vi "Target CSM.vi"(5 "Init State(\"Macro: Initialize\")":string="Macro: Initialize", 7 "Name (\"\" to Use UUID)":string="CSM Tiny") -> ()   [LabVIEW 2017]
doc: "Template for building CSM Module without User Interface.\n\n<b>Inputs:</b>\n- <b>Name (\"\" to Use UUID)</b>: Module Name\n - If Input is \"\", an uuid will be used for module name. The module is marked as stand-alone mode and will not be included in module list.\n - Fi Input end with '#', the module will worked in worker mode. Modules with the same name will shared the same message queue. Any external message will be processed by one of the modules, depends on who is free.\n - Otherwise, the input string will be used as module name, which should be unique in system. CSM will go to \"Critical Error\" state if duplicated module name is used in system.\n\n<b>Outputs:</b>\n - N/A"
uses:
  src/user.lib/_NEVSTOP/Communicable State Machine(CSM)/AdvanceAPI/CSM - Revert Arguments-Safe String.vi
  src/user.lib/_NEVSTOP/Communicable State Machine(CSM)/AdvanceAPI/CSM - Break Down Multiple States String.vi
  src/user.lib/_NEVSTOP/Communicable State Machine(CSM)/AdvanceAPI/CSM - Compact Multiple States.vi
  src/user.lib/_NEVSTOP/Communicable State Machine(CSM)/AdvanceAPI/CSM - Make String Arguments Safe.vi
  src/user.lib/_NEVSTOP/Communicable State Machine(CSM)/AdvanceAPI/CSM - Keywords.vi
  src/user.lib/_NEVSTOP/Communicable State Machine(CSM)/_Shared/Trim Single-line Text.vi
  src/user.lib/_NEVSTOP/Communicable State Machine(CSM)/Communicable State Machine.lvlib
panel:
  out "Error Occurred":errorcluster
  out "State History":string
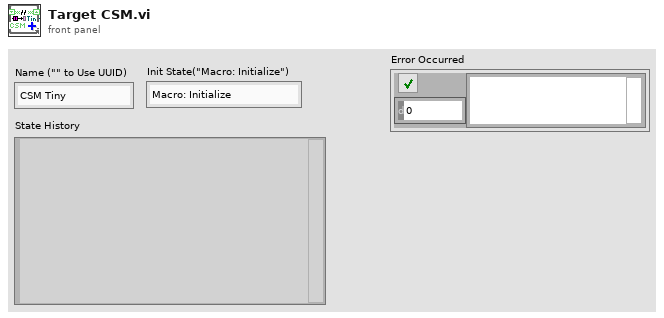
[diagram p1: front panel]
types:
  T1 = enum32{"Invalid", "Standard", "Closed", "Hidden", "Minimized", "Maximized"}
  T2 = enum32{"invalid app kind", "Development System", "Run Time System", "Student Edition", "Embedded LabVIEW", "Evaluation", "Custom"}
  T3 = typedef "Communicable State Machine.lvlib/_CSM_Response Source Message.ctl" = cluster{"‘State":string, "’Arguments":string, "’Error":errorcluster}
  T4 = cluster{"Current VI Reference":refnum<vi>, "Close Panel on Exit?":bool}
  T5 = cluster{"Core":cluster{"Current VI Reference":refnum<vi>, "Close Panel on Exit?":bool}, "Your Boolean data":bool, "Your string data":string}
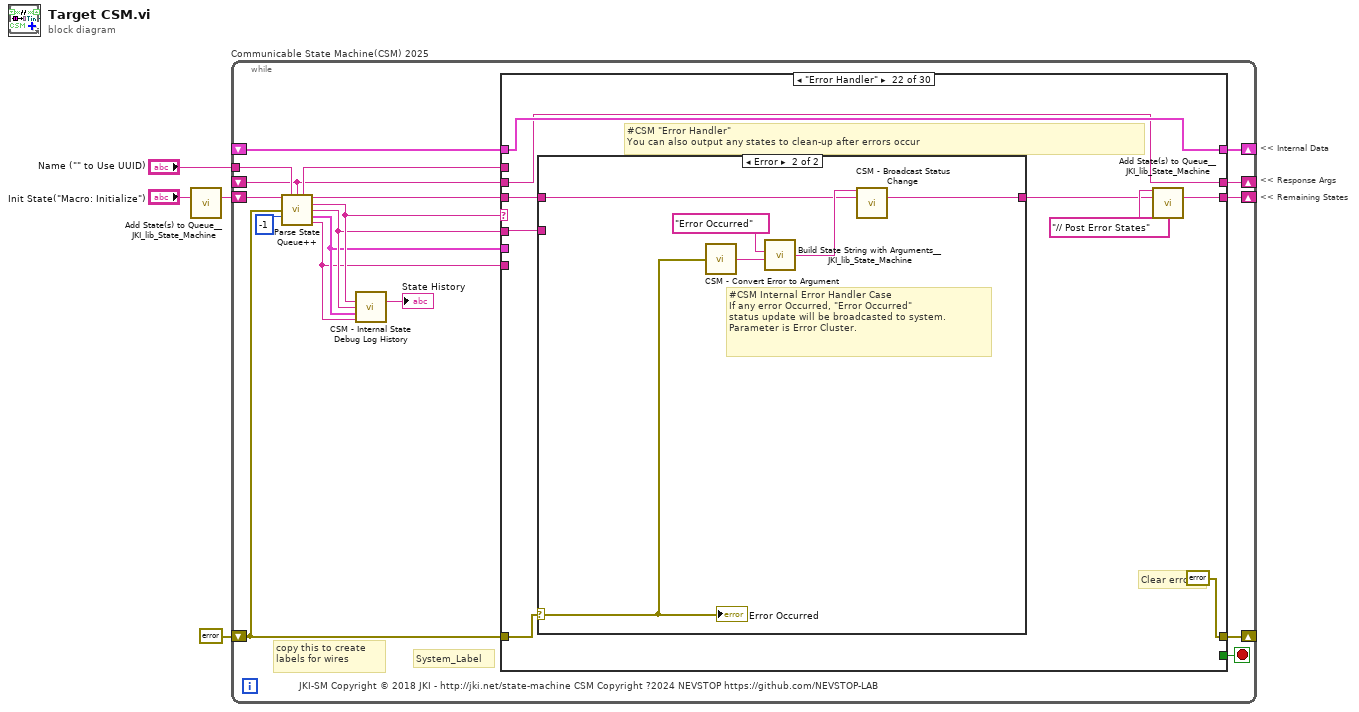
[diagram p0: block diagram]
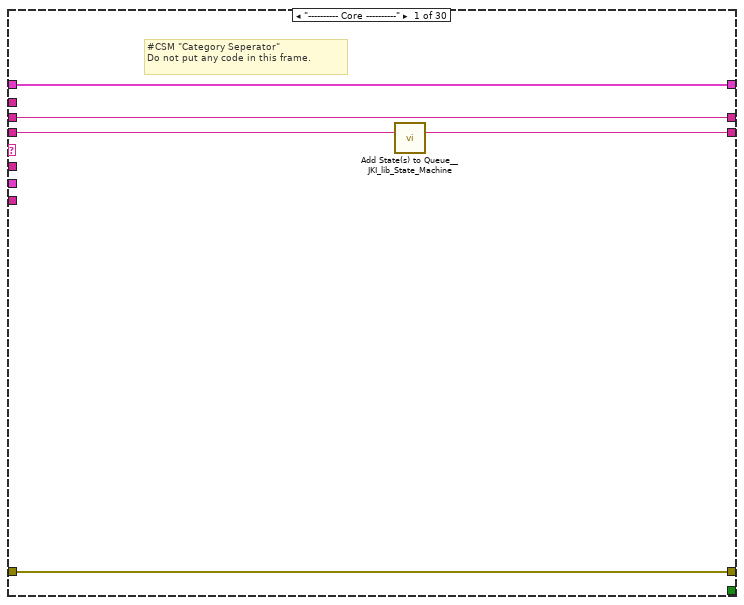
[diagram p2: hidden frame]
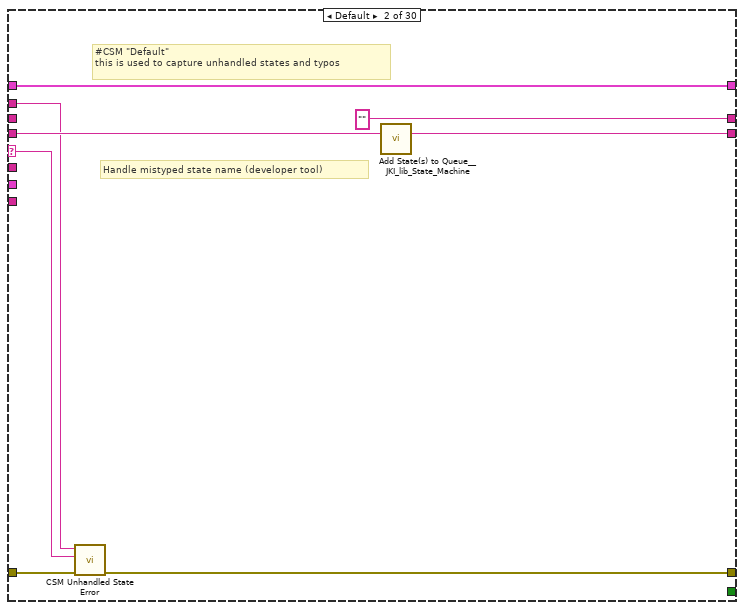
[diagram p3: hidden frame]
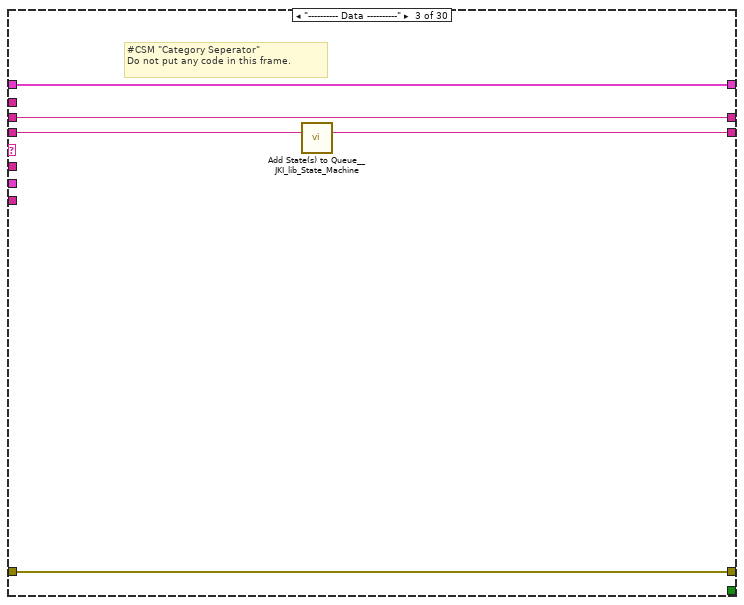
[diagram p4: hidden frame]
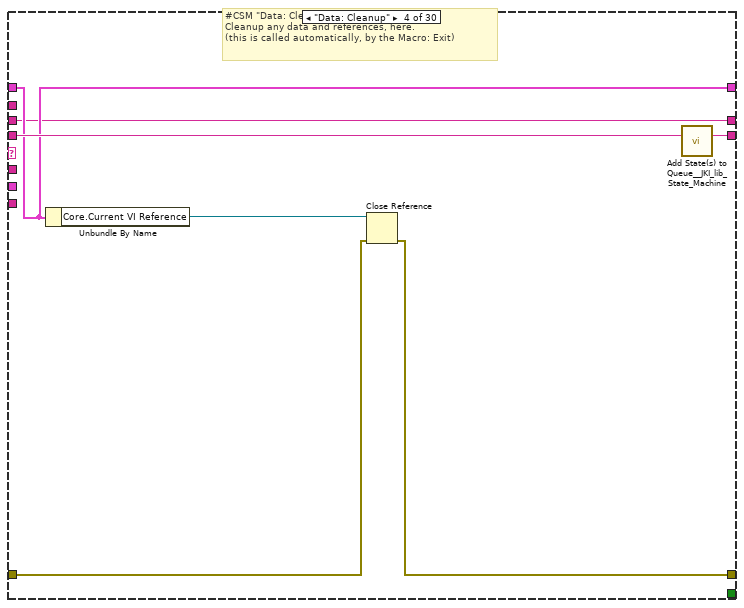
[diagram p5: hidden frame]
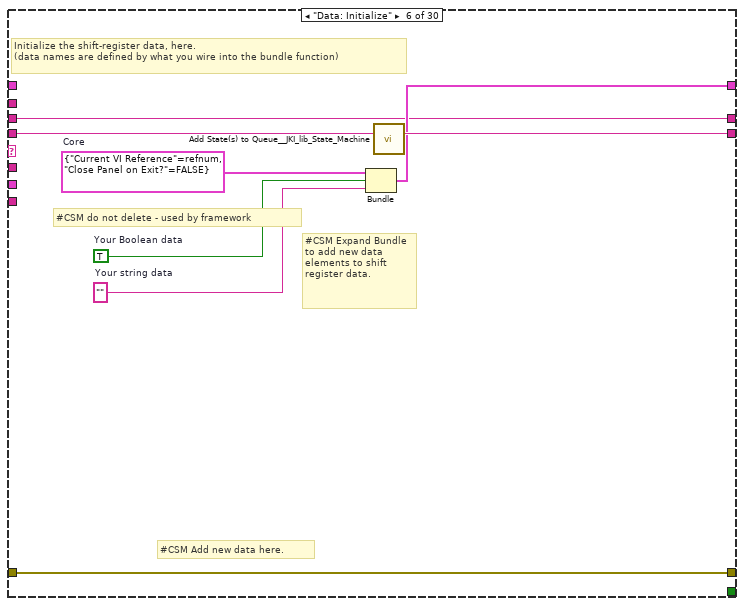
[diagram p7: hidden frame]
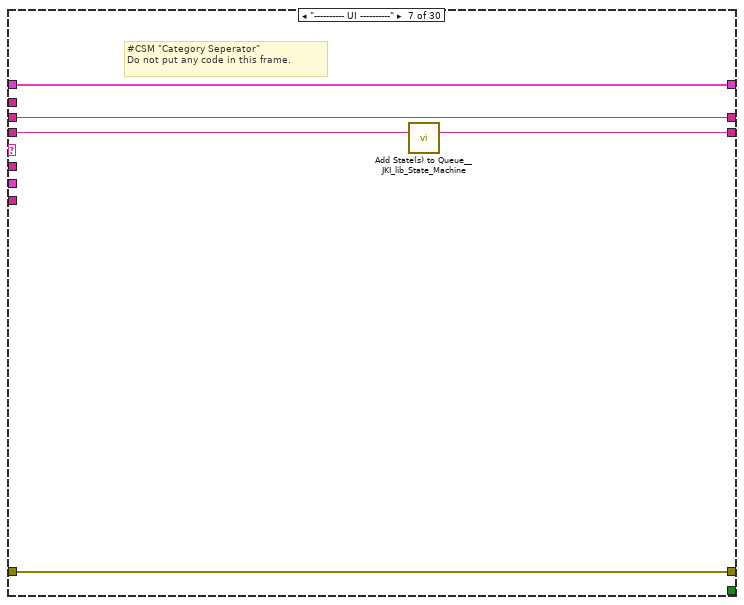
[diagram p8: hidden frame]
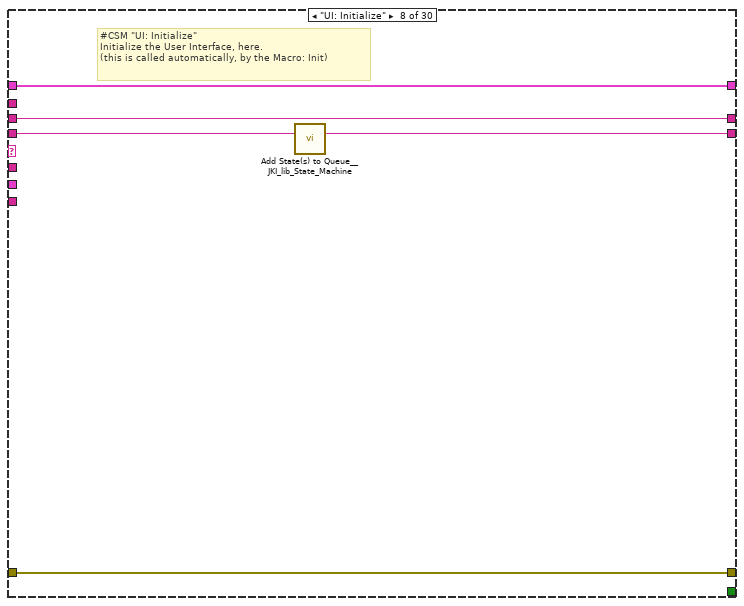
[diagram p9: hidden frame]
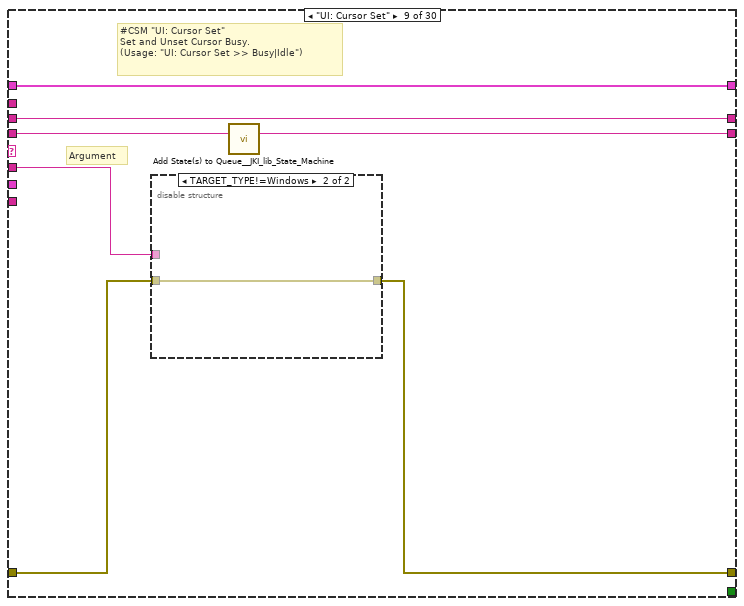
[diagram p10: hidden frame]
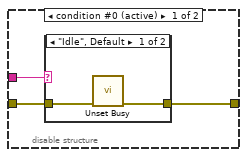
[diagram p11: hidden frame]
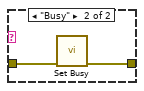
[diagram p12: hidden frame]
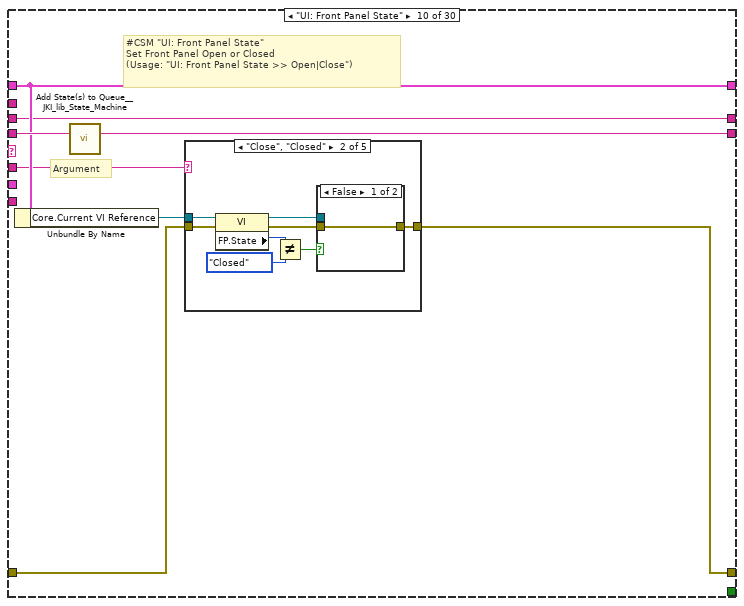
[diagram p13: hidden frame]
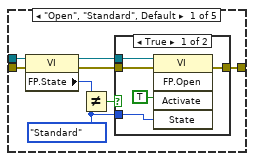
[diagram p14: hidden frame]
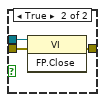
[diagram p16: hidden frame]
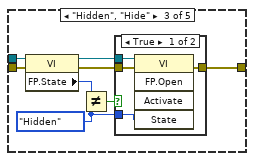
[diagram p17: hidden frame]
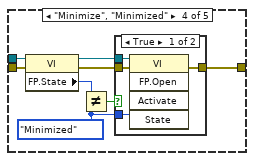
[diagram p19: hidden frame]
diagram:
  # "<< Internal Data"
  # "<< Response Args"
  # "<< Remaining States"
  n1 = call <vilib>:"Add State(s) to Queue__JKI_lib_State_Machine.vi"("State(s) in (\"\")"="Init State(\"Macro: Initialize\")") -> ("States Out"=w4:string)  [unwired: 14 in]
  n2 = while "Communicable State Machine(CSM) 2025" {
    shift-right: [w17] -> _
    shift-left: _ -> [w16]
    shift-right: [w20] -> _
    shift-left: errorcluster {"status"=FALSE, "code"=0, "source"=""} ("error out") -> [w15]
    shift-right: [w19] -> _
    shift-left: w4 -> [w21]
    tunnel: "Name (\"\" to Use UUID)" -> [w13]
    shift-right: [w14] -> _
    shift-left: _ -> [w7]
    stop <- w18 stop-if-true
    # "copy this to create labels for wires"
    # "System_Label"
    # "JKI-SM Copyright © 2018 JKI - http://jki.net/state-machine CSM Copyright ?2024 NEVSTOP https://github.com/NEVSTOP-LAB"
    n3 = call "Parse State Queue++.vi"("State Queue"=w21, "Name (\"\" to Use UUID)"=w13, "Response Arguments"=w7, "Previous Error"=w15, "Dequeue (1 ms)"=-1 ("Timeout")) -> ("Name Used"=w8:string, "Remaining States"=w22:string, "Current State"=w12:string, "Arguments"=w11:string, "Additional Information"=w10:T3, "Source CSM"=w9:string)  [unwired: 5 in]
    n4 = call "CSM - Internal State Debug Log History.vi"("State"=w12, "Arguments (\"\")"=w11, ">> Response Source Message >>"=w10, "Source (\"\")"=w9) -> ("Debug Log"=→"State History":string)  [unwired: 11 in]
    n5 = case shown="\"Error Handler\"" w12 {
      selector: w12 -> [_ w30 _ _ _ _ _ _ _ _ _ _ _ _ _ _ _ _ _ _ _ _ _ _ _ _ _ _ _ _]
      tunnel: w22 -> [w27 w34 w40 w47 w50 w59 w64 w69 w76 w92 w162 w170 w176 w179 w183 w189 w196 w201 w206 w209 w213 w219 w240 w247 w254 w265 w281 w289 w304 w310]
      tunnel: w11 -> [_ _ _ _ _ _ _ _ w71 w86 _ _ _ _ w185 _ _ _ _ _ _ w218 w239 w246 w253 w260 w276 _ _ _]
      tunnel: w16 -> [w24 w32 w37 w43 w51 _ w61 w67 w74 w88 w159 w165 w173 w178 w184 w190 w193 w199 w204 w210 w214 w216 w234 w242 w249 w263 w279 w290 w298 w308]
      tunnel: [w25 w28 w38 w44 w49 w56 w62 w66 w72 w89 w160 w164 w172 w180 w182 w188 w194 w198 w203 w208 w212 errorcluster {"status"=FALSE, "code"=0, "source"=""} ("error out") w236 w244 w251 w266 w282 w288 w292 w307] -> w20
      tunnel: w15 -> [w25 w35 w38 w45 w49 w56 w62 w66 w73 w90 w160 w164 w172 w180 w182 w188 w194 w198 w203 w208 w212 w217 w237 w245 w252 _ _ w288 w292 w307]
      tunnel: [w26 w33 w39 w42 w50 w58 w63 w68 w75 w91 w161 w169 w175 w179 w183 w189 w195 w200 w205 w209 w213 w220 w235 w243 w250 w264 w280 w289 w303 w309] -> w19
      tunnel: [_ _ _ _ _ _ _ _ _ _ _ _ _ _ _ _ _ _ _ _ _ _ _ _ _ _ _ _ _ TRUE] -> w18
      tunnel: [w24 w32 w37 w43 w51 w57 w61 w67 w74 w88 w159 w165 w173 w178 w184 w190 w193 w199 w204 w210 w214 w216 w234 w242 w249 w262 w278 w290 w302 w308] -> w17
      tunnel: w9 -> [_ _ _ _ _ _ _ _ _ _ _ _ _ _ _ _ _ _ _ _ _ _ _ _ _ w261 w277 _ _ _]
      tunnel: w10 -> [_ _ _ _ _ _ _ _ _ _ _ _ _ _ _ _ _ _ _ _ _ _ _ _ _ w256 w272 _ _ _]
      tunnel: [w23 "" w36 w41 w48 w52 w60 w65 w70 w85 w158 w163 w171 w177 w181 "API1 Response" w192 w197 w202 w207 w211 w215 w233 w241 w248 w255 w271 w287 w291 w306] -> w14
      tunnel: w8 -> [_ w29 _ _ _ _ _ _ _ _ _ _ _ _ _ _ _ _ _ _ _ _ w238 _ _ _ _ _ _ _]
      tunnel: w7 -> [w23 _ w36 w41 w48 w52 w60 w65 w70 w85 w158 w163 w171 w177 w181 _ w192 w197 w202 w207 w211 w215 w233 w241 w248 w255 w271 w287 w291 w306]
      frame "---------- Core ----------" {
        # "#CSM \"Category Seperator\"\nDo not put any code in this frame."
        n6 = call <vilib>:"Add State(s) to Queue__JKI_lib_State_Machine.vi"("State(s) in (\"\")"=w27) -> ("States Out"=w26:string)  [unwired: 14 in]
      }
      frame Default {
        # "#CSM \"Default\"\nthis is used to capture unhandled states and typos"
        # "Handle mistyped state name (developer tool)"
        n7 = call "CSM Unhandled State Error.vi"("error in (no error)"=w35, "Undefined State"=w30, "CSM Name"=w29) -> ("error out"=w28:errorcluster)  [unwired: 8 in]
        n8 = call <vilib>:"Add State(s) to Queue__JKI_lib_State_Machine.vi"("State(s) in (\"\")"=w34) -> ("States Out"=w33:string)  [unwired: 14 in]
      }
      frame "---------- Data ----------" {
        # "#CSM \"Category Seperator\"\nDo not put any code in this frame."
        n9 = call <vilib>:"Add State(s) to Queue__JKI_lib_State_Machine.vi"("State(s) in (\"\")"=w40) -> ("States Out"=w39:string)  [unwired: 14 in]
      }
      frame "Data: Cleanup" {
        # "#CSM \"Data: Cleanup\"\nCleanup any data and references, here.\n(this is called automatically, by the Macro: Exit)"
        n10 = Unbundle By Name(w43) -> ("Core.Current VI Reference"=w46:refnum<vi>)
        n11 = Close Reference(reference=w46, error in (no error)=w45) -> (error out=w44:errorcluster)
        n12 = call <vilib>:"Add State(s) to Queue__JKI_lib_State_Machine.vi"("State(s) in (\"\")"=w47) -> ("States Out"=w42:string)  [unwired: 14 in]
      }
      frame "Data: Update Indicators" {
      }
      frame "Data: Initialize" {
        w53 = T4 {"Current VI Reference"=refnum, "Close Panel on Exit?"=FALSE}  # Core
        w55 = TRUE  # Your Boolean data
        w54 = ""  # Your string data
        # "#CSM do not delete - used by framework"
        # "#CSM Expand Bundle to add new data elements to shift register data."
        # "#CSM Add new data here."
        # "Initialize the shift-register data, here.\n(data names are defined by what you wire into the bundle function)"
        n13 = Bundle("Core"=w53, "Your Boolean data"=w55, "Your string data"=w54) -> (w57:T5)  [unwired: 1 in]
        n14 = call <vilib>:"Add State(s) to Queue__JKI_lib_State_Machine.vi"("State(s) in (\"\")"=w59) -> ("States Out"=w58:string)  [unwired: 14 in]
      }
      frame "---------- UI ----------" {
        # "#CSM \"Category Seperator\"\nDo not put any code in this frame."
        n15 = call <vilib>:"Add State(s) to Queue__JKI_lib_State_Machine.vi"("State(s) in (\"\")"=w64) -> ("States Out"=w63:string)  [unwired: 14 in]
      }
      frame "UI: Initialize" {
        # "#CSM \"UI: Initialize\"\nInitialize the User Interface, here.\n(this is called automatically, by the Macro: Init)"
        n16 = call <vilib>:"Add State(s) to Queue__JKI_lib_State_Machine.vi"("State(s) in (\"\")"=w69) -> ("States Out"=w68:string)  [unwired: 14 in]
      }
      frame "UI: Cursor Set" {
        # "#CSM \"UI: Cursor Set\"\nSet and Unset Cursor Busy.\n(Usage: \"UI: Cursor Set >> Busy|Idle\")"
        # "Argument"
        n17 = disable-structure shown="TARGET_TYPE!=Windows" {
          disable-tunnel: w73 -> [w79 w84]
          disable-tunnel: [w78 w84] -> w72
          disable-tunnel: w71 -> [w77 _]
          frame condition #0 (active) {
            n18 = case shown="\"Idle\", Default" w77 {
              tunnel: w79 -> [w81 w83]
              tunnel: [w80 w82] -> w78
              frame "Idle", Default {
                n19 = call <vilib>:"Unset Busy.vi"("error in (no error)"=w81) -> ("error out"=w80:errorcluster)  [unwired: 10 in]
              }
              frame "Busy" {
                n20 = call <vilib>:"Set Busy.vi"("error in (no error)"=w83) -> ("error out"=w82:errorcluster)  [unwired: 9 in, 1 out]
              }
            }
          }
          frame condition #1 {
          }
        }
        n21 = call <vilib>:"Add State(s) to Queue__JKI_lib_State_Machine.vi"("State(s) in (\"\")"=w76) -> ("States Out"=w75:string)  [unwired: 14 in]
      }
      frame "UI: Front Panel State" {
        # "#CSM \"UI: Front Panel State\"\nSet Front Panel Open or Closed\n(Usage: \"UI: Front Panel State >> Open|Close\")"
        # "Argument"
        n22 = Unbundle By Name(w88) -> ("Core.Current VI Reference"=w87:refnum<vi>)
        n23 = call <vilib>:"Add State(s) to Queue__JKI_lib_State_Machine.vi"("State(s) in (\"\")"=w92) -> ("States Out"=w91:string)  [unwired: 14 in]
        n24 = case shown="\"Close\", \"Closed\"" w86 {
          tunnel: w90 -> [w98 w113 w124 w137 w150]
          tunnel: [w100 w114 w126 w139 w152] -> w89
          tunnel: w87 -> [w99 w111 w125 w138 w151]
          frame "Open", "Standard", Default {
            w93 = T1."Standard" ("State")
            n25 = property class="VI"(reference=w99, error in=w98) -> (reference out=w96:refnum<vi>, error out=w97:errorcluster, "FP.State"=w95:T1)
            n26 = Not Equal?(x=w95, y=w93) -> (x != y?=w94:bool)
            n27 = case shown="True" w94 {
              tunnel: [w104 w106] -> w100
              tunnel: w97 -> [w103 w106]
              tunnel: w96 -> [w102 _]
              tunnel: w93 -> [w101 _]
              frame True {
                n28 = invoke class="VI" method="FP.Open"(reference=w102, error in=w103, "Activate"=TRUE, "State"=w101) -> (error out=w104:errorcluster)  [unwired: 1 in, 4 out]
              }
              frame False {
              }
            }
          }
          frame "Close", "Closed" {
            n29 = property class="VI"(reference=w111, error in=w113) -> (reference out=w110:refnum<vi>, error out=w112:errorcluster, "FP.State"=w108:T1)
            n30 = Not Equal?(x=w108, y=T1."Closed" ("Front Panel Window:State")) -> (x != y?=w107:bool)
            n31 = case shown="False" w107 {
              tunnel: [w115 w118] -> w114
              tunnel: w112 -> [w115 w117]
              tunnel: w110 -> [_ w116]
              frame False {
              }
              frame True {
                n32 = invoke class="VI" method="FP.Close"(reference=w116, error in=w117) -> (error out=w118:errorcluster)  [unwired: 1 in, 2 out]
              }
            }
          }
          frame "Hidden", "Hide" {
            w119 = T1."Hidden" ("State")
            n33 = property class="VI"(reference=w125, error in=w124) -> (reference out=w122:refnum<vi>, error out=w123:errorcluster, "FP.State"=w121:T1)
            n34 = Not Equal?(x=w121, y=w119) -> (x != y?=w120:bool)
            n35 = case shown="True" w120 {
              tunnel: [w130 w131] -> w126
              tunnel: w123 -> [w129 w131]
              tunnel: w122 -> [w128 _]
              tunnel: w119 -> [w127 _]
              frame True {
                n36 = invoke class="VI" method="FP.Open"(reference=w128, error in=w129, "State"=w127) -> (error out=w130:errorcluster)  [unwired: 2 in, 4 out]
              }
              frame False {
              }
            }
          }
          frame "Minimize", "Minimized" {
            w132 = T1."Minimized" ("State")
            n37 = property class="VI"(reference=w138, error in=w137) -> (reference out=w135:refnum<vi>, error out=w136:errorcluster, "FP.State"=w134:T1)
            n38 = Not Equal?(x=w134, y=w132) -> (x != y?=w133:bool)
            n39 = case shown="True" w133 {
              tunnel: [w143 w144] -> w139
              tunnel: w136 -> [w142 w144]
              tunnel: w135 -> [w141 _]
              tunnel: w132 -> [w140 _]
              frame True {
                n40 = invoke class="VI" method="FP.Open"(reference=w141, error in=w142, "State"=w140) -> (error out=w143:errorcluster)  [unwired: 2 in, 4 out]
              }
              frame False {
              }
            }
          }
          frame "Maximize", "Maximized" {
            w145 = T1."Maximized" ("State")
            n41 = property class="VI"(reference=w151, error in=w150) -> (reference out=w148:refnum<vi>, error out=w149:errorcluster, "FP.State"=w147:T1)
            n42 = Not Equal?(x=w147, y=w145) -> (x != y?=w146:bool)
            n43 = case shown="True" w146 {
              tunnel: [w156 w157] -> w152
              tunnel: w149 -> [w155 w157]
              tunnel: w148 -> [w154 _]
              tunnel: w145 -> [w153 _]
              frame True {
                n44 = invoke class="VI" method="FP.Open"(reference=w154, error in=w155, "State"=w153) -> (error out=w156:errorcluster)  [unwired: 2 in, 4 out]
              }
              frame False {
              }
            }
          }
        }
      }
      frame "---------- Macro ----------" {
        # "#CSM \"Category Seperator\"\nDo not put any code in this frame."
        n45 = call <vilib>:"Add State(s) to Queue__JKI_lib_State_Machine.vi"("State(s) in (\"\")"=w162) -> ("States Out"=w161:string)  [unwired: 14 in]
      }
      frame "Macro: Exit" {
        # "#CSM \"Macro: Exit\"\nExit Macro (This is called once, when the VI exits)"
        n46 = call <vilib>:"Add State(s) to Queue__JKI_lib_State_Machine.vi"("State(s) in Front (\"\")"="//Exit Sub-Modules ", "State(s) at Back (\"\")"="Data: Cleanup\nExit") -> ("States Out"=w167:string)  [unwired: 13 in]
        n47 = call <vilib>:"Add State(s) to Queue__JKI_lib_State_Machine.vi"("State(s) in Front (\"\")"=w167, "State(s) in (\"\")"=w170) -> ("States Out"=w169:string)  [unwired: 13 in]
      }
      frame "Macro: Initialize" {
        # "#CSM \"Macro: Initialize\"\nInitialization Macro (This is called once, when the VI starts)"
        n48 = call <vilib>:"Add State(s) to Queue__JKI_lib_State_Machine.vi"("State(s) in Front (\"\")"="Data: Initialize\nInitialize Core Data\nData: Update Indicators", "State(s) in (\"\")"=w176) -> ("States Out"=w175:string)  [unwired: 13 in]
      }
      frame "---------- API ----------" {
        # "#CSM \"Category Seperator\"\nDo not put any code in this frame."
      }
      frame "API: API2" {
        # "#CSM API Example\nCopy/Rename this case for your own API"
        # "unpack Hex String  to Variant\nif complex parameter is needed."
        n49 = call "CSM - Convert HexStr to Data.vi"("HEX String"=w185) -> ()  [unwired: 7 in, 2 out]
        n50 = disable-structure shown="Enabled" {
          disable-tunnel: [w186 "API2 Response"] -> _
          frame Disabled {
            # "pack variant to hexstr \nif complex response is needed."
            # "complex Response"
            n51 = call "CSM - Convert Data to HexStr.vi"() -> ("HEX String (0-9,A-F)"=w186:string)  [unwired: 9 in]
          }
          frame Enabled {
          }
        }
      }
      frame "API: API1" {
        # "#CSM API Example\nCopy/Rename this case for your own API"
        # "#CSM >> Msg/Rep's CSM >>\nIf you need to tell who triggered this state , use this string. If it's this case itself, this string is \"\"."
        # "#CSM >> Arguments >>\nDeal with the parameter if any"
        # "#CSM Response\nConnect this to return the response of your API"
      }
      frame "---------- Action ----------" {
        # "#CSM \"Category Seperator\"\nDo not put any code in this frame."
        n52 = call <vilib>:"Add State(s) to Queue__JKI_lib_State_Machine.vi"("State(s) in (\"\")"=w196) -> ("States Out"=w195:string)  [unwired: 14 in]
      }
      frame "Action: action2" {
        # "#CSM \"Internal State\"\nThis category is used for holding internal states"
        n53 = call <vilib>:"Add State(s) to Queue__JKI_lib_State_Machine.vi"("State(s) in (\"\")"=w201) -> ("States Out"=w200:string)  [unwired: 14 in]
      }
      frame "Action: action1" {
        # "#CSM \"Internal State\"\nThis category is used for holding internal states"
        n54 = call <vilib>:"Add State(s) to Queue__JKI_lib_State_Machine.vi"("State(s) in (\"\")"=w206) -> ("States Out"=w205:string)  [unwired: 14 in]
      }
      frame "Idle" {
        (unwired) refnum<file> refnum ("refnum out")
        # "#CSM \"Idle/Event Handler\"\nexecutes when the state queue is empty"
      }
      frame "CSM Documentation" {
        # "#CSM Documentation"
        # "#CSM State Syntax\n\n// Comment line, all text to the right of “//” will be ignored\n// Local Message Example\nDoSth: DoA >> Arguments\n\n// Sync Call Example\nAPI: xxxx >> Arguments -@ TargetModule\n\n// Async Call Example\nAPI: xxxx >> Arguments -> TargetModule\n\n// Async Call without Reply Example\nAPI: xxxx >> Arguments ->| TargetModule\n\n// Broadcast normal status:\nStatus >> StatusArguments  -><status>\n\n// Broadcast Interrupt status:\nInterrupt >> StatusArguments  -><interrupt>\n\n// Register Source Module's status to Handler Module\nStatus@Source Module >> Handler Module@Handler Module -><register>\n\n// Unegister Source Module's status\nStatus@Source Module >> Handler Module -><unregister>"
        # "#CSM README FIRST\n\nCommunicable State Machine(CSM) is a LabVIEW application framework that builds upon JKI State Machine(JKISM). It follows the pattern of JKISM and extends the keywords to describe message communication between modules, including concepts such as Sync-Message, Async-Message, Subscription/Unsubscription of status - essential elements for creating reusable code modules. For more information, please visit the CSM wiki: https://nevstop-lab.github.io/CSM-Wiki/\n\nFor instructions on JKI State Machine, visit: \n    http://jki.net/state-machine/\nFor information about CSM, visit: \n    https://github.com/NEVSTOP-LAB"
        # "#CSM \"Documentation\"\nCase for holding CSM Documenation"
      }
      frame "Error Handler" {
        # "#CSM \"Error Handler\"\nYou can also output any states to clean-up after errors occur"
        # "Clear error"
        n55 = case shown="Error" w217 {
          selector: w217 -> [_ w227]
          tunnel: [w226 w229] -> w221
          tunnel: w219 -> [w226 w228]
          tunnel: w218 -> [w225 _]
          frame No Error {
            n56 = call "CSM - Convert Argument to Error.vi"("Argument"=w225) -> ("Error"=w224:errorcluster)  [unwired: 4 in]
            n57 = flat-sequence {
              tunnel: w224 -> [_]
              frame #0 {
                # "#CSM External Error Handler Case\nUsually, it's because This CSM register others' \"Error Occurred\" status with \"Error Handler\". If other CSM have any error, the error will be passed here for central handling."
              }
            }
          }
          frame Error {
            # "#CSM Internal Error Handler Case \nIf any error Occurred, \"Error Occurred\" \nstatus update will be broadcasted to system.\nParameter is Error Cluster."
            n58 = call "CSM - Convert Error to Argument.vi"("Error"=w227) -> ("Argument"=w231:string)  [unwired: 4 in]
            n59 = call <vilib>:"Build State String with Arguments__JKI_lib_State_Machine.vi"("Arguments (\"\")"=w231, "State"="Error Occurred" ("Status with Arguments")) -> ("State with Arguments"=w230:string)  [unwired: 4 in]
            n60 = call "CSM - Broadcast Status Change.vi"("Status With Arguments"=w230, "State Queue"=w228) -> ("Remaining States"=w229:string)  [unwired: 13 in]
            "Error Occurred" <- w227
          }
        }
        n61 = call <vilib>:"Add State(s) to Queue__JKI_lib_State_Machine.vi"("State(s) in Front (\"\")"="// Post Error States", "State(s) in (\"\")"=w221) -> ("States Out"=w220:string)  [unwired: 13 in]
      }
      frame "Critical Error" {
        (unwired) TRUE
        # "#CSM \"Critical Error\"\nWhen any un-recoverable error occurs, CSM goes into this case."
        # "#CSM Stop in Critical Error\nWhen Critical Error occurs, Stop the loop immediately. Do NOT change this unless you fully understand the impact."
        n62 = call "CSM Critical Error.vi"("error in (no error)"=w237, "Arugments (As Reason)"=w239, "CSM Name"=w238) -> ("error out"=w236:errorcluster)  [unwired: 8 in]
        n63 = call <vilib>:"Add State(s) to Queue__JKI_lib_State_Machine.vi"("State(s) in (\"\")"=w240) -> ("States Out"=w235:string)  [unwired: 14 in]
      }
      frame "Target Timeout Error" {
        # "#CSM \"Target Timeout Error\"\nWhen This CSM could not get the sync-call response in time, This CSM goes into this case."
        n64 = call "CSM Target Timeout Error.vi"("error in (no error)"=w245, "Arguments (As CSM Name)"=w246) -> ("error out"=w244:errorcluster)  [unwired: 9 in]
        n65 = call <vilib>:"Add State(s) to Queue__JKI_lib_State_Machine.vi"("State(s) in (\"\")"=w247) -> ("States Out"=w243:string)  [unwired: 14 in]
      }
      frame "Target Error" {
        # "#CSM \"Target Error\"\nWhen This CSM try to communicate with an un-existed CSM, This CSM goes into this case."
        n66 = call "CSM Target Error.vi"("error in (no error)"=w252, "Arguments (As CSM Name)"=w253) -> ("error out"=w251:errorcluster)  [unwired: 9 in]
        n67 = call <vilib>:"Add State(s) to Queue__JKI_lib_State_Machine.vi"("State(s) in (\"\")"=w254) -> ("States Out"=w250:string)  [unwired: 14 in]
      }
      frame "Async Response" {
        n68 = Unbundle(w256) -> ("‘State"=w259:string, "’Arguments"=w258:string, "’Error"=w257:errorcluster)
        n69 = case shown="Default" w259 {
          tunnel: [w267] -> w264
          tunnel: w265 -> [w268]
          tunnel: [w270] -> w262
          tunnel: w263 -> [w270]
          tunnel: [w269] -> w266
          tunnel: w257 -> [w269]
          tunnel: w261 -> [_]
          tunnel: w260 -> [_]
          tunnel: w258 -> [_]
          frame Default {
            # "#CSM \"Async Response\"\nHandle Async-call Response (\"Async Response\" for ->)"
            # "#CSM \"Response\"\nHandle Sync-call Response (\"Response\" for -@)"
            # "#CSM Response Comments\nAfter Message is executed, CSM goes to this state for receive the response.\n    For Async Message(->), \"Async Response\" is used. This CSM will goes to \"Async Message Posted\" immediately and receive the \"Async Response\" after the callee finishes the message.\n    For Sync Message(@),  This CSM will wait until the message is done and immediately goes to \"Response\""
            n70 = call <vilib>:"Add State(s) to Queue__JKI_lib_State_Machine.vi"("State(s) in (\"\")"=w268) -> ("States Out"=w267:string)  [unwired: 14 in]
          }
        }
      }
      frame "Response" {
        n71 = Unbundle(w272) -> ("‘State"=w275:string, "’Arguments"=w274:string, "’Error"=w273:errorcluster)
        n72 = case shown="Default" w275 {
          tunnel: [w283] -> w280
          tunnel: w281 -> [w284]
          tunnel: [w286] -> w278
          tunnel: w279 -> [w286]
          tunnel: [w285] -> w282
          tunnel: w273 -> [w285]
          tunnel: w277 -> [_]
          tunnel: w276 -> [_]
          tunnel: w274 -> [_]
          frame Default {
            # "#CSM \"Async Response\"\nHandle Async-call Response (\"Async Response\" for ->)"
            # "#CSM \"Response\"\nHandle Sync-call Response (\"Response\" for -@)"
            # "#CSM Response Comments\nAfter Message is executed, CSM goes to this state for receive the response.\n    For Async Message(->), \"Async Response\" is used. This CSM will goes to \"Async Message Posted\" immediately and receive the \"Async Response\" after the callee finishes the message.\n    For Sync Message(@),  This CSM will wait until the message is done and immediately goes to \"Response\""
            n73 = call <vilib>:"Add State(s) to Queue__JKI_lib_State_Machine.vi"("State(s) in (\"\")"=w284) -> ("States Out"=w283:string)  [unwired: 14 in]
          }
        }
      }
      frame "Async Message Posted" {
        # "#CSM \"Async Message Posted\"\nAfter Async Message is posted (-> or ->| ), CSM goes to this state for post-action.\nYou can use Argument - State to tell which Async Message is called."
      }
      frame "Initialize Core Data" {
        # "#CSM \"Initialize Core Data\"\nThis is used to determine panel behavior on exit"
        # "originally closed?"
        # "exe?"
        # "If panel starts closed or is an EXE, then close it when we exit"
        n74 = control-ref of="Current VI Reference"() -> (w296:refnum<vi>)
        n75 = property class="VI"() -> ("FP.State"=w295:T1)  [unwired: 2 in, 2 out]
        n76 = property class="App"() -> ("App.Kind"=w301:T2)  [unwired: 2 in, 2 out]
        n77 = Equal?(x=w295, y=T1."Closed" ("Front Panel Window:State")) -> (x = y?=w293:bool)
        n78 = Equal?(x=w301, y=T2."Run Time System" ("Application:Kind")) -> (x = y?=w299:bool)
        n79 = Or(x=w293, y=w299) -> (x .or. y?=w297:bool)
        n80 = Bundle By Name(cluster=w298, "Core.Current VI Reference"=w296, "Core.Close Panel on Exit?"=w297) -> (w302:T5)
        n81 = call <vilib>:"Add State(s) to Queue__JKI_lib_State_Machine.vi"("State(s) in (\"\")"=w304) -> ("States Out"=w303:string)  [unwired: 14 in]
      }
      frame "Exit" {
        # "#CSM \"Exit\"\nCase for exiting the loop. No errors that occur here will be handled."
        n82 = call <vilib>:"Add State(s) to Queue__JKI_lib_State_Machine.vi"("State(s) in (\"\")"=w310) -> ("States Out"=w309:string)  [unwired: 14 in]
      }
    }
  }
